vi "ConnectDL_vi.vi"(8 "error in (no error)":errorcluster, 9 "Command":string, 10 "ON/OFF":bool, 11 "Control in":refnum<class "Control-Server.lvclass">) -> (0 "error out":errorcluster, 3 "Control out":refnum<class "Control-Server.lvclass">)   [LabVIEW 2015, in "Control-Server.lvclass"]
uses:
  Control-Server.lvclass
  dependecies/ControlsVIs/Clusters-def/Message types.ctl
  Control-Server.lvclass/Control-Server.ctl
  Delay Line/DelayLine.lvclass
  Message/Message.lvclass
  GeneralFunctionality/GeneralFunctionality.lvclass
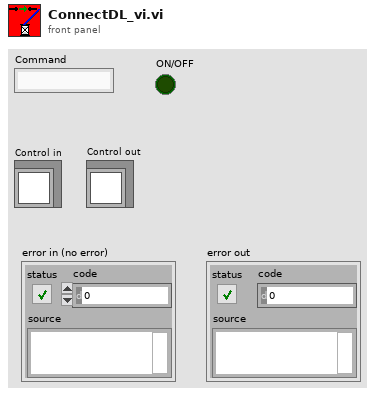
[diagram p1: front panel]
types:
  T1 = typedef "Message types.ctl" = string
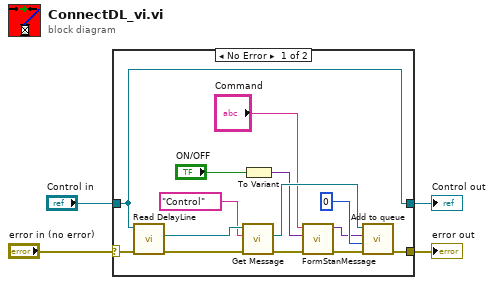
[diagram p0: block diagram]
diagram:
  n1 = case shown="No Error" "error in (no error)" {
    selector: "error in (no error)" -> [w9 w20]
    tunnel: [w15 w19] -> w4
    tunnel: "Control in" -> [w15 w19]
    tunnel: [w8 w20] -> w2
    frame No Error {
      n2 = call "Read DelayLine.vi"("error in (no error)"=w9, "Control in"=w15) -> ("error out"=w16:errorcluster, "DelayLine.lvclass"=w17:refnum<class "DelayLine.lvclass">)  [unwired: 7 in, 1 out]
      n3 = call "Get Message.vi"("error in (no error)"=w16, "Message type"=T1 "Control", "GeneralFunctionality en entrée"=w17) -> ("error out"=w6:errorcluster, "Message.lvclass"=w18:refnum<class "Message.lvclass">)  [unwired: 6 in, 1 out]
      n4 = To Variant(anything="ON/OFF") -> (Variant=w10:variant)
      n5 = call "FormStanMessage.vi"("error in"=w6, "data"=w10, "Command"="Command") -> ("error out"=w7:errorcluster, "message"=w11:variant)  [unwired: 7 in]
      n6 = call "Add to queue.vi"("error in (no error)"=w7, "timeout in ms (-1)"=0, "Data"=w11, "Message in"=w18) -> ("error out"=w8:errorcluster)  [unwired: 6 in, 1 out]
    }
    frame Error {
    }
  }
  "error out" <- w2
  "Control out" <- w4
